vi "Test Initial Verify.vi"() -> ()   [LabVIEW 2020, in "Basic.Mechanics.Tests.lvclass"]
uses:
  Basic.Mechanics.Tests.lvclass
  Source/Approval Tests/Options/Options.lvclass
  Source/Approval Tests/Report Nothing/Report Nothing.lvclass
  C:/Users/SAS/Desktop/ApprovalTests.LabVIEW/Source/Approval Tests/Reporter/Reporter.lvclass
  Source/Approval Tests/Options/Options.lvclass/Options.ctl
  Source/Approval Tests/Naming Data/Naming Data.lvclass/Naming Data.ctl
  d27a92d8-1944-4452-9057-093efe2cb2fc.vi
  Source/Approval Tests/Options/Write Reporter.vi
  Source/Approval Tests/Verify Core.vi
  d27a92d8-1944-4452-9057-093efe2cb2fc.vi/93c5622b-9fb7-41e0-8c76-3fde37e94e34.vi
  Source/Approval Tests/Update Test Name if Not Defined.vi
  Source/Approval Tests/Options/Read Scrubber.vi
  Source/Approval Tests/Options/Read Namer.vi
  Source/Approval Tests/Options/Read Naming Data.vi
  Source/Approval Tests/Options/Read Reporter.vi
  d27a92d8-1944-4452-9057-093efe2cb2fc.vi/93c5622b-9fb7-41e0-8c76-3fde37e94e34.vi/04cb982b-2eda-40d0-8d7e-90f8e0b569b2.vi
  Source/Approval Tests/Naming Data/Read Test VI Name.vi
  Source/Approval Tests/Naming Data/Write Test VI Name.vi
  Source/Approval Tests/Options/Add Label to Namer.vi
  Source/Approval Tests/conv EOL.vi
  <vilib>/Utility/libraryn.llb/Check if File or Folder Exists.vi
  Source/Approval Tests/Reporter/Report.vi
  <vilib>/addons/_JKI Toolkits/Caraya/classes/Assert/Assert False.vi
  <vilib>/addons/_JKI Toolkits/Caraya/classes/Assert/Assert Equal Value_Variant.vi
  Source/Approval Tests/Scrubber/Scrubber.lvclass
  Source/Approval Tests/Namer/Namer.lvclass
  Source/Approval Tests/Naming Data/Naming Data.lvclass
  Source/Approval Tests/Reporter/Reporter.lvclass
  <vilib>/addons/_JKI Toolkits/Caraya/classes/Test/Test.lvclass
  <vilib>/addons/_JKI Toolkits/Caraya/classes/Assert/Assert.lvclass
panel:
  out "error out":errorcluster
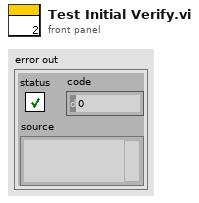
[diagram p1: front panel]
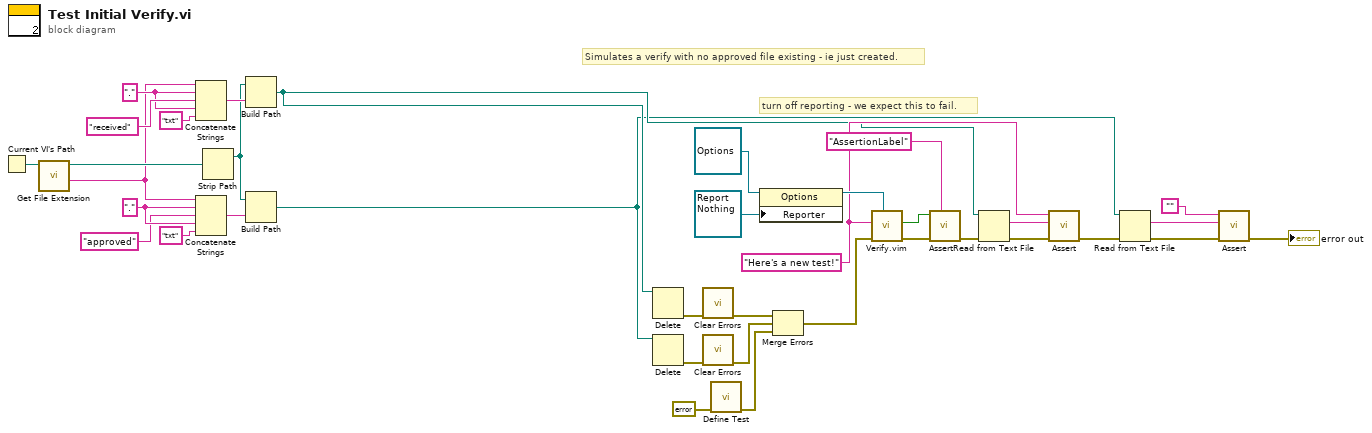
[diagram p0: block diagram]
diagram:
  w11 = "." ("string")
  w16 = "." ("string")
  w8 = "Here's a new test!"
  # "turn off reporting - we expect this to fail."
  # "Simulates a verify with no approved file existing - ie just created."
  n1 = Current VI's Path() -> (path=w18:path)
  n2 = call <vilib>:"Get File Extension.vi"("file"=w18) -> ("filename without extension"=w10:string, "dup file"=w17:path)  [unwired: 6 in, 3 out]
  n3 = Concatenate Strings(w10, w11, "received" ("string"), w11, "txt" ("string")) -> (w13:string)
  n4 = Concatenate Strings(w10, w16, "approved" ("string"), w16, "txt" ("string")) -> (w14:string)
  n5 = Strip Path(path=w17) -> (stripped path=w5:path)  [unwired: 1 out]
  n6 = Build Path(base path=w5, name or relative path=w13) -> (appended path=w2:path)
  n7 = Build Path(base path=w5, name or relative path=w14) -> (appended path=w1:path)
  n8 = Delete(path (use dialog)=w2) -> (error out=w30:errorcluster)  [unwired: 4 in, 2 out]
  n9 = Delete(path (use dialog)=w1) -> (error out=w29:errorcluster)  [unwired: 4 in, 2 out]
  n10 = call <vilib>:"Clear Errors.vi"("error in (no error)"=w30) -> ("error out"=w28:errorcluster)  [unwired: 5 in, 1 out]
  n11 = call <vilib>:"Clear Errors.vi"("error in (no error)"=w29) -> ("error out"=w27:errorcluster)  [unwired: 5 in, 1 out]
  n12 = call <vilib>:"Define Test.vi"("error in (no error)"=errorcluster {"status"=FALSE, "code"=0, "source"=""}) -> ("error out"=w24:errorcluster)  [unwired: 9 in, 1 out]
  n13 = property on="Property Node" class="Options"(reference=refnum<class "Options.lvclass"> refnum ("Options"), "Reporter"=refnum<class "Report Nothing.lvclass"> refnum ("Approval Tests.lvlib:Report Nothing")) -> (reference out=w22:refnum<class "Options.lvclass">)  [unwired: 1 in, 1 out]
  n14 = Merge Errors(w28, w27, w24) -> (w26:errorcluster)
  n15 = call "Verify.vim"("Options"=w22, "error in"=w26, "Anything"=w8) -> ("error out"=w25:errorcluster, "Passed?"=w19:bool)  [unwired: 6 in, 1 out]
  n16 = call-poly <vilib>:"Assert.vi"("Label"="AssertionLabel" ("Label (VI Title)"), "error in (no error)"=w25, "False?"=w19) -> ("error out"=w35:errorcluster)  [unwired: 7 in, 1 out]
  n17 = Read from Text File(file (use dialog)=w2, error in=w35) -> (text=w9:string, error out=w34:errorcluster)  [unwired: 2 in, 2 out]
  n18 = call-poly <vilib>:"Assert.vi"("error in (no error)"=w34, "Y"=w9, "X"=w8) -> ("error out"=w33:errorcluster)  [unwired: 7 in, 1 out]
  n19 = Read from Text File(file (use dialog)=w1, error in=w33) -> (text=w7:string, error out=w32:errorcluster)  [unwired: 2 in, 2 out]
  n20 = call-poly <vilib>:"Assert.vi"("error in (no error)"=w32, "Y"=w7, "X"="") -> ("error out"=→"error out":errorcluster)  [unwired: 7 in, 1 out]
